vi "ai_act.vi"(8 "empty rounds":u32, 9 "live rounds":u32, 11 "difficulty":u32) -> (2 "item num":u32, 3 "use item":bool, 4 "shoot self":bool, 10 "Items":i32[](array[numeric]))   [LabVIEW 2025]
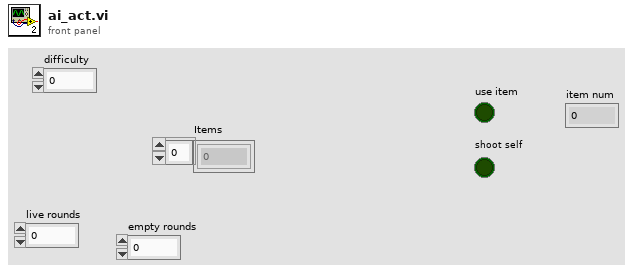
[diagram p1: front panel]
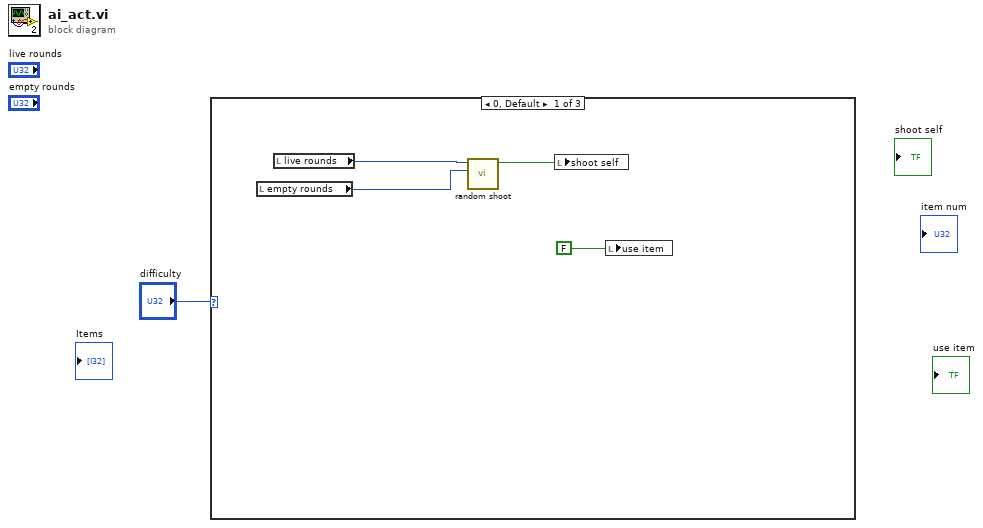
[diagram p0: block diagram]
diagram:
  n1 = case shown="0, Default" "difficulty" {
    frame 0, Default {
      n2 = local read "empty rounds"() -> (w3:u32)
      n3 = local read "live rounds"() -> (w4:u32)
      n4 = call "random shoot.vi"("empty rounds"=w3, "live rounds"=w4) -> ("hit self"=w5:bool)  [unwired: 9 in]
      n5 = local write "shoot self"(w5) -> ()
      n6 = local write "use item"(FALSE) -> ()
    }
    frame 1 {
    }
    frame 2 {
    }
  }
